vi "spilib_open.vi"(8 "error in (no error)":errorcluster, 10 "SPI Bus":T1) -> (0 "error out":errorcluster, 3 "handle out":i32)   [LabVIEW 2017]
uses:
  <vilib>/Rock Robotics/SystemInterfaces/spilib/spi_bus.ctl
  <vilib>/Utility/error.llb/Error Cluster From Error Code.vi
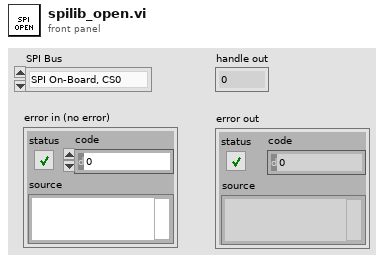
[diagram p1: front panel]
types:
  T1 = typedef "spi_bus.ctl" = enum16{"SPI On-Board, CS0", "SPI On-Board, CS1", "SPI On-Board, CS2", "SPI On-Board, CS3", "SPI MXP", "Invalid"}
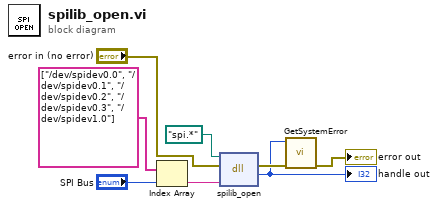
[diagram p0: block diagram]
diagram:
  n1 = Index Array(array=string[] ["/dev/spidev0.0", "/dev/spidev0.1", "/dev/spidev0.2", "/dev/spidev0.3", "/dev/spidev1.0"], index="SPI Bus") -> (element=w8:string)
  n2 = dll-call lib="?" fn="spilib_open"(path in=path "spi.*", error in="error in (no error)", "device"=w8) -> (error out=w4:errorcluster, "handle"=w3:i32)  [unwired: 2 in, 1 out]
  "handle out" <- w3
  n3 = call <vilib>:"GetSystemError.vi"("error in (no error)"=w4, "Retval"=w3) -> ("error out"=→"error out":errorcluster)  [unwired: 9 in]
